vi "Command (write) - EP.vi"(7 "timeout ms (100)":i32=100, 8 "error in (no error)":errorcluster, 9 "Encoder Position":i32=-2147483648, 10 "IP":string, 11 "connection ID in":refnum<k16>) -> (0 "error out":errorcluster, 3 "connection ID out":refnum<k16>)   [LabVIEW 2016, in "SMD-7615.lvlib" / "eSCL.lvlib"]
doc: "EP - Encoder Position\nThe EP command allows the host to define the present encoder position. For example, if the encoder is at 4500 counts, and you would like to refer to this position as 0, send EP0. To ensure that the internal position counter resets properly, use SP immediately following EP. For example, to set the position to zero after a homing routine, send EP0 then SP0."
uses:
  eSCL.lvlib
  I32 Command and Param.ctl
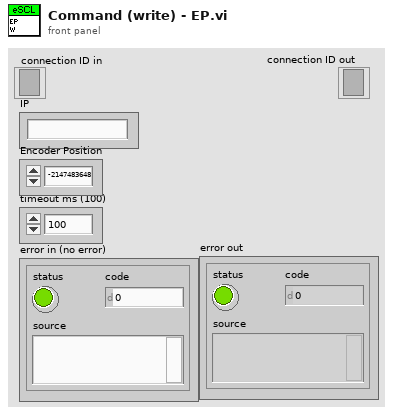
[diagram p1: front panel]
types:
  T1 = typedef "SMD-7615.lvlib/eSCL.lvlib/I32 Command and Param.ctl" = cluster{"Command":string, "I32 Parameler":i32, "I32 Parameler Default":i32, "I32 Parameler Coerece Upper":i32, "I32 Parameler Coerece Lower":i32}
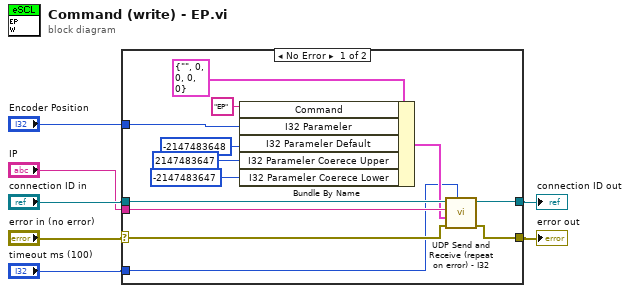
[diagram p0: block diagram]
diagram:
  n1 = case shown="No Error" "error in (no error)" {
    selector: "error in (no error)" -> [w12 w21]
    tunnel: "connection ID in" -> [w15 w22]
    tunnel: [w10 w22] -> w2
    tunnel: [w9 w21] -> w1
    tunnel: "IP" -> [w14 _]
    tunnel: "timeout ms (100)" -> [w11 _]
    tunnel: "Encoder Position" -> [w16 _]
    frame No Error {
      n2 = Bundle By Name(cluster=T1 {"Command"="", "I32 Parameler"=0, "I32 Parameler Default"=0, "I32 Parameler Coerece Upper"=0, "I32 Parameler Coerece Lower"=0} ("I32 Command & Param"), "Command"="EP", "I32 Parameler"=w16, "I32 Parameler Default"=-2147483648 ("DBL Parameler Default"), "I32 Parameler Coerece Upper"=2147483647 ("DBL Parameler Coerece Upper"), "I32 Parameler Coerece Lower"=-2147483647 ("DBL Parameler Coerece Lower")) -> (w13:T1)
      n3 = call "UDP Send and Receive (repeat on error) - I32.vi"("timeout ms (100)"=w11, "error in (no error)"=w12, "I32 Command & Param"=w13, "IP"=w14, "connection ID in"=w15) -> ("error out"=w9:errorcluster, "connection ID out"=w10:refnum<k16>)  [unwired: 4 in, 1 out]
    }
    frame Error {
    }
  }
  "connection ID out" <- w2
  "error out" <- w1
